vi "NMR_Short_RF_Pulse_Sequence_V1.vi"() -> ()   [LabVIEW 2020]
uses:
  <instrlib>/niFgen/niFgen.llb/niFgen Waveform Type.ctl
  <instrlib>/niFgen/niFgen.llb/niFgen_ctl Trigger DigEdge - Edge Values (Ring).ctl
  <instrlib>/niFgen/niFgen.llb/niFgen_ctl Trigger Source Values (Ring).ctl
  <instrlib>/niFgen/niFgen.llb/niFgen Output Mode.ctl
  <instrlib>/niFgen/niFgen.llb/niFgen Trigger Mode.ctl
  <instrlib>/niFgen/niFgen.llb/niFgen Configure Digital Edge Start Trigger.vi
  <instrlib>/niFgen/niFgen.llb/niFgen Create Waveform (I16).vi
panel:
  in  "Sample Rate":dbl=50000000.0 format="%.2p"
  in  "Frequency":dbl=27500000.0 format="%.4p"
  in  "Delay Time (ms)":u32=4000
  in  "Number of Scans":i32=1
  in  "DC Offset":dbl(knob) scale=-0.5..0.5 scale format="%#.1f"
  in  "Gain":dbl(knob)=1.3 min=0.0 max=5.0 scale=0.0..5.0 scale format="%#.1f"
  in  "FGEN Resource Name 2":refnum<k15>="FGEN1" caption="FGEN Resource Name"
  in  "Waveform Information Array":T1(array[cluster])=[{"Waveform Type"=7, "Amplitude"=0.0, "# of points"=1000}, {"Waveform Type"=7, "Amplitude"=1.0, "# of points"=1200}, {"Waveform Type"=7, "Amplitude"=0.0, "# of points"=250000}, {"Waveform Type"=7, "Amplitude"=1.0, "# of points"=2400}, {"Waveform Type"=7, "Amplitude"=0.0, "# of points"=500000}, {"Waveform Type"=7, "Amplitude"=0.0, "# of points"=4000}, {"Waveform Type"=7, "Amplitude"=0.0, "# of points"=500000}, {"Waveform Type"=7, "Amplitude"=0.0, "# of points"=4000}, {"Waveform Type"=7, "Amplitude"=0.0, "# of points"=500000}, {"Waveform Type"=7, "Amplitude"=0.0, "# of points"=4000}, {"Waveform Type"=7, "Amplitude"=0.0, "# of points"=10000000}] {"Amplitude" min=0.0 max=1.0 format="%.2f"; "Waveform Type" items=["Sine", "Cosine", "Triangle", "Square", "Sawtooth", "Increasing Ramp", "Decreasing Ramp", "DC Value"]}
  in  "Amplitude":dbl=0.35 format="%0_3g"
  in  "FGEN Resource Name":refnum<k15>="Dev1"
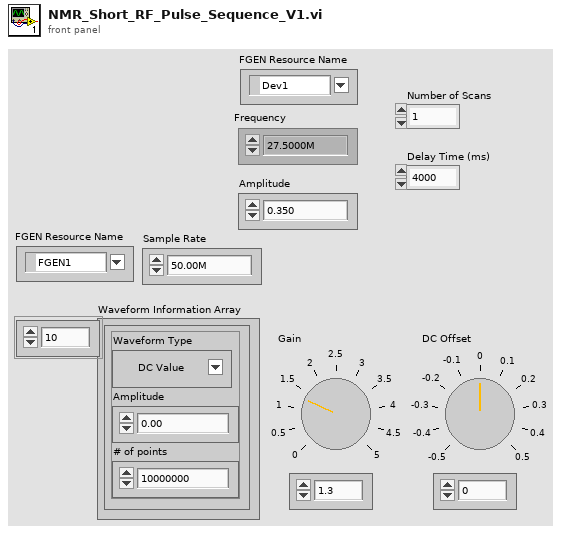
[diagram p1: front panel]
types:
  T1 = cluster{"Waveform Type":u16, "Amplitude":dbl, "# of points":u32}[]
  T2 = typedef "niFgen_ctl Trigger Source Values (Ring).ctl" = string
  T3 = typedef "niFgen Trigger Mode.ctl" = i32
  T4 = typedef "niFgen Output Mode.ctl" = u32
  T5 = typedef "niFgen_ctl Trigger DigEdge - Edge Values (Ring).ctl" = i32
  T6 = typedef "niFgen Waveform Type.ctl" = i32
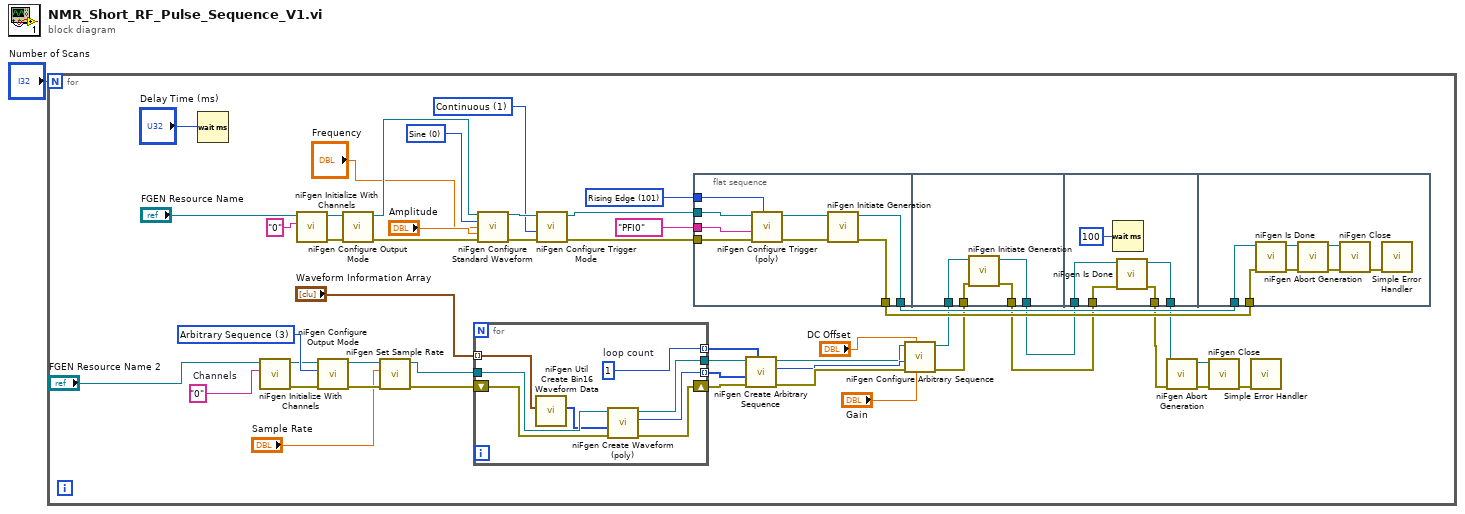
[diagram p0: block diagram]
diagram:
  n1 = for {
    N: "Number of Scans" -> [_]
    w13 = T3 1 items=["Single", "Continuous", "Stepped", "Burst"] ("Trigger Mode (default: 1=continuous)")
    w16 = "0"  # Channels
    w25 = T4 3 items=["Standard Function", "Frequency List", "Arbitrary Waveform", "Arbitrary Sequence", "Script"] ("output mode")
    w39 = T5 101 items=["Rising Edge"=101, "Falling Edge"=102] ("Edge (Rising)")
    w41 = T6 0 items=["Sine", "Square", "Triangle", "Ramp Up", "Ramp Down", "DC", "Noise", "User"] ("Waveform")
    n2 = Wait (ms)(milliseconds to wait="Delay Time (ms)") -> ()  [unwired: 1 out]
    n3 = call <instrlib>:"niFgen Initialize With Channels.vi"("Channel Name"=w16, "Resource Name"="FGEN Resource Name 2") -> ("error out"=w19:errorcluster, "Instrument Handle Out"=w18:refnum<k15>)  [unwired: 8 in]
    n4 = call <instrlib>:"niFgen Initialize With Channels.vi"("Channel Name"="0", "Resource Name"="FGEN Resource Name") -> ("error out"=w46:errorcluster, "Instrument Handle Out"=w49:refnum<k15>)  [unwired: 8 in]
    n5 = call <instrlib>:"niFgen Configure Output Mode.vi"("error in (no error)"=w19, "Output Mode (default: 0=Standard Function)"=w25, "Instrument Handle"=w18) -> ("error out"=w3:errorcluster, "Instrument Handle Out"=w6:refnum<k15>)  [unwired: 6 in]
    n6 = call <instrlib>:"niFgen Configure Output Mode.vi"("error in (no error)"=w46, "Instrument Handle"=w49) -> ("error out"=w45:errorcluster, "Instrument Handle Out"=w48:refnum<k15>)  [unwired: 7 in]
    n7 = call <instrlib>:"niFgen Set Sample Rate.vi"("error in (no error)"=w3, "Sample Rate (Samp/s)"="Sample Rate", "Instrument Handle"=w6) -> ("error out"=w4:errorcluster, "Instrument Handle Out"=w5:refnum<k15>)  [unwired: 7 in]
    n8 = for {
      shift-right: [w56] -> w26
      shift-left: w4 -> [w54]
      tunnel: [w57] -> w27
      tunnel: w5 -> [w55]
      tunnel: [w53] -> w28 mode=indexing
      tunnel: "Waveform Information Array" -> [w51] mode=indexing
      tunnel: [w50] -> w23 mode=indexing
      w50 = 1  # loop count
      n9 = call <instrlib>:"niFgen Util Create Bin16 Waveform Data.vi"("Waveform"=w51) -> ("Waveform Data"=w52:i16[])  [unwired: 10 in]
      n10 = call-poly <instrlib>:"niFgen Create Waveform (poly).vi"("error in (no error)"=w54, "Waveform Data Array"=w52, "Instrument Handle"=w55) -> ("error out"=w56:errorcluster, "Waveform Handle"=w53:i32, "Instrument Handle Out"=w57:refnum<k15>)  [unwired: 6 in]
    }
    n11 = call <instrlib>:"niFgen Configure Standard Waveform.vi"("Instrument Handle"=w48, "Waveform"=w41, "Frequency"="Frequency", "Amplitude"="Amplitude", "error in (no error)"=w45) -> ("Instrument Handle Out"=w47:refnum<k15>, "error out"=w44:errorcluster)  [unwired: 9 in]
    n12 = call <instrlib>:"niFgen Configure Trigger Mode.vi"("error in (no error)"=w44, "Trigger Mode (default: 1=continuous)"=w13, "Instrument Handle"=w47) -> ("error out"=w38:errorcluster, "Instrument Handle Out"=w36:refnum<k15>)  [unwired: 7 in]
    n13 = flat-sequence {
      tunnel: w39 -> [w64]
      tunnel: w38 -> [w63]
      tunnel: T2 "PFI0" ("Source") -> [w62]
      tunnel: w36 -> [w61]
      tunnel: [w60] -> w34
      tunnel: [w59] -> w35
      tunnel: w15 -> [w69]
      tunnel: w14 -> [w68]
      tunnel: [w67] -> w11
      tunnel: [w66] -> w10
      tunnel: w11 -> [w73]
      tunnel: w10 -> [w72]
      tunnel: [w71] -> w9
      tunnel: [w70] -> w8
      tunnel: w35 -> [w76]
      tunnel: w34 -> [w75]
      frame #0 {
        n14 = call-poly <instrlib>:"niFgen Configure Trigger (poly).vi"("Edge (Rising)"=w64, "error in (no error)"=w63, "Source"=w62, "Instrument Handle"=w61) -> ("error out"=w58:errorcluster, "Instrument Handle Out"=w65:refnum<k15>)  [unwired: 6 in]
        n15 = call <instrlib>:"niFgen Initiate Generation.vi"("error in (no error)"=w58, "Instrument Handle"=w65) -> ("error out"=w59:errorcluster, "Instrument Handle Out"=w60:refnum<k15>)  [unwired: 8 in]
      }
      frame #1 {
        n16 = call <instrlib>:"niFgen Initiate Generation.vi"("error in (no error)"=w69, "Instrument Handle"=w68) -> ("error out"=w67:errorcluster, "Instrument Handle Out"=w66:refnum<k15>)  [unwired: 8 in]
      }
      frame #2 {
        n17 = Wait (ms)(milliseconds to wait=u32 100) -> ()  [unwired: 1 out]
        n18 = call <instrlib>:"niFgen Is Done.vi"("error in (no error)"=w73, "Instrument Handle"=w72) -> ("error out"=w71:errorcluster, "Instrument Handle Out"=w70:refnum<k15>)  [unwired: 7 in, 1 out]
      }
      frame #3 {
        n19 = call <instrlib>:"niFgen Is Done.vi"("error in (no error)"=w76, "Instrument Handle"=w75) -> ("error out"=w79:errorcluster, "Instrument Handle Out"=w78:refnum<k15>)  [unwired: 7 in, 1 out]
        n20 = call <instrlib>:"niFgen Abort Generation.vi"("error in (no error)"=w79, "Instrument Handle"=w78) -> ("error out"=w80:errorcluster, "Instrument Handle Out"=w81:refnum<k15>)  [unwired: 8 in]
        n21 = call <instrlib>:"niFgen Close.vi"("error in (no error)"=w80, "Instrument Handle"=w81) -> ("error out"=w77:errorcluster)  [unwired: 9 in]
        n22 = call <vilib>:"Simple Error Handler.vi"("error in (no error)"=w77) -> ()  [unwired: 4 in, 5 out]
      }
    }
    n23 = call <instrlib>:"niFgen Create Arbitrary Sequence.vi"("Loop Counts Array"=w23, "error in (no error)"=w26, "Waveform Handles Array"=w28, "Instrument Handle"=w27) -> ("error out"=w31:errorcluster, "Sequence Handle"=w30:i32, "Instrument Handle Out"=w29:refnum<k15>)  [unwired: 5 in]
    n24 = call <instrlib>:"niFgen Configure Arbitrary Sequence.vi"("Gain"="Gain", "Offset"="DC Offset", "error in (no error)"=w31, "Sequence Handle"=w30, "Instrument Handle"=w29) -> ("error out"=w15:errorcluster, "Instrument Handle Out"=w14:refnum<k15>)  [unwired: 5 in]
    n25 = call <instrlib>:"niFgen Abort Generation.vi"("error in (no error)"=w9, "Instrument Handle"=w8) -> ("error out"=w32:errorcluster, "Instrument Handle Out"=w33:refnum<k15>)  [unwired: 8 in]
    n26 = call <instrlib>:"niFgen Close.vi"("error in (no error)"=w32, "Instrument Handle"=w33) -> ("error out"=w24:errorcluster)  [unwired: 9 in]
    n27 = call <vilib>:"Simple Error Handler.vi"("error in (no error)"=w24) -> ()  [unwired: 4 in, 5 out]
  }
